vi "CmdExe.Callback for .NET OutputDataRecieved Event, EnQ StdOutData.vi"(4 "QStdOut":refnum<queue>, 5 "Event Data":cluster{"sender":refnum<k24>, "e":refnum<k24>}, 6 "Control Ref":refnum<k24>, 7 "Event Common Data":T1) -> ()   [LabVIEW 2024]
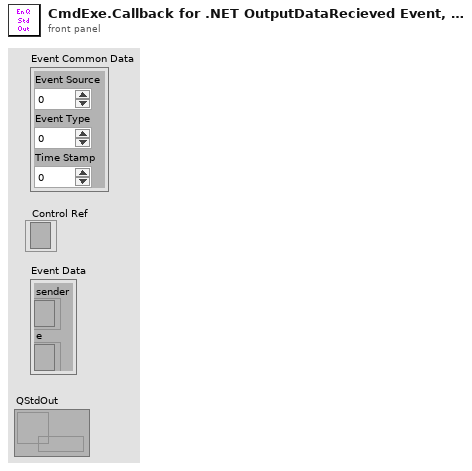
[diagram p1: front panel]
types:
  T1 = cluster{"Event Source":i32, "Event Type":u32, "Time Stamp":u32}
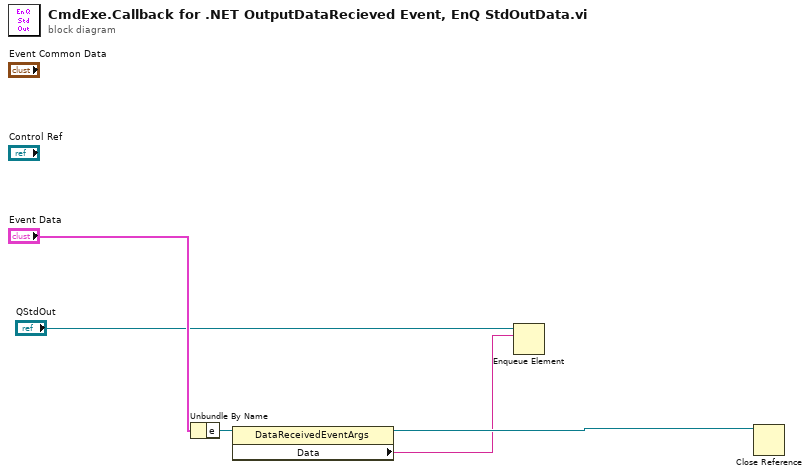
[diagram p0: block diagram]
diagram:
  n1 = Unbundle By Name("Event Data") -> ("e"=w4:refnum<k24>)
  n2 = property class="DataReceivedEventArgs"(reference=w4) -> (reference out=w3:refnum<k24>, "Data"=w1:string)  [unwired: 1 in, 1 out]
  n3 = Enqueue Element(queue="QStdOut", element=w1) -> ()  [unwired: 2 in, 3 out]
  n4 = Close Reference(reference=w3) -> ()  [unwired: 1 in, 1 out]
